vi "Dimmer BaseStation.vi"() -> ()   [LabVIEW 2014, in "ESP8266 WiFi Wrapper.lvlib"]
uses:
  ESP8266 WiFi Wrapper.lvlib
  <vilib>/Aledyne-TSXperts/Arduino Compatible Compiler for LabVIEW/Arduino Compatible Compiler for LabVIEW.lvlib
panel:
  in  "DNS address":u8[](array[numeric])=[1, 2, 3, 4]
  in  "IP address":u8[](array[numeric])=[192, 168, 0, 42]
  in  "Gateway":u8[](array[numeric])=[192, 168, 0, 1]
  in  "Subnet mask":u8[](array[numeric])=[255, 255, 255, 0]
  in  "Password":string="12345678"
  in  "SSID":string="ESP8266 Wifi Example"
  in  "Listen Port":u8=80
  in  "error in (no error)":errorcluster
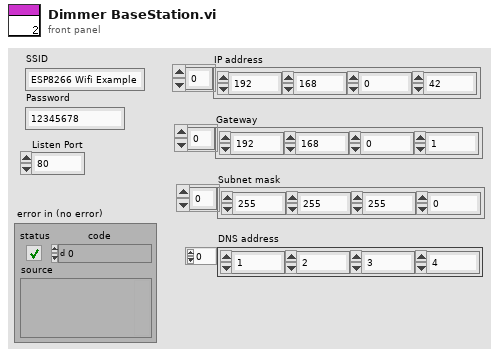
[diagram p1: front panel]
types:
  T1 = enum16{"WIFI_OFF", "WIFI_STA", "WIFI_AP", "WIFI_AP_STA"}
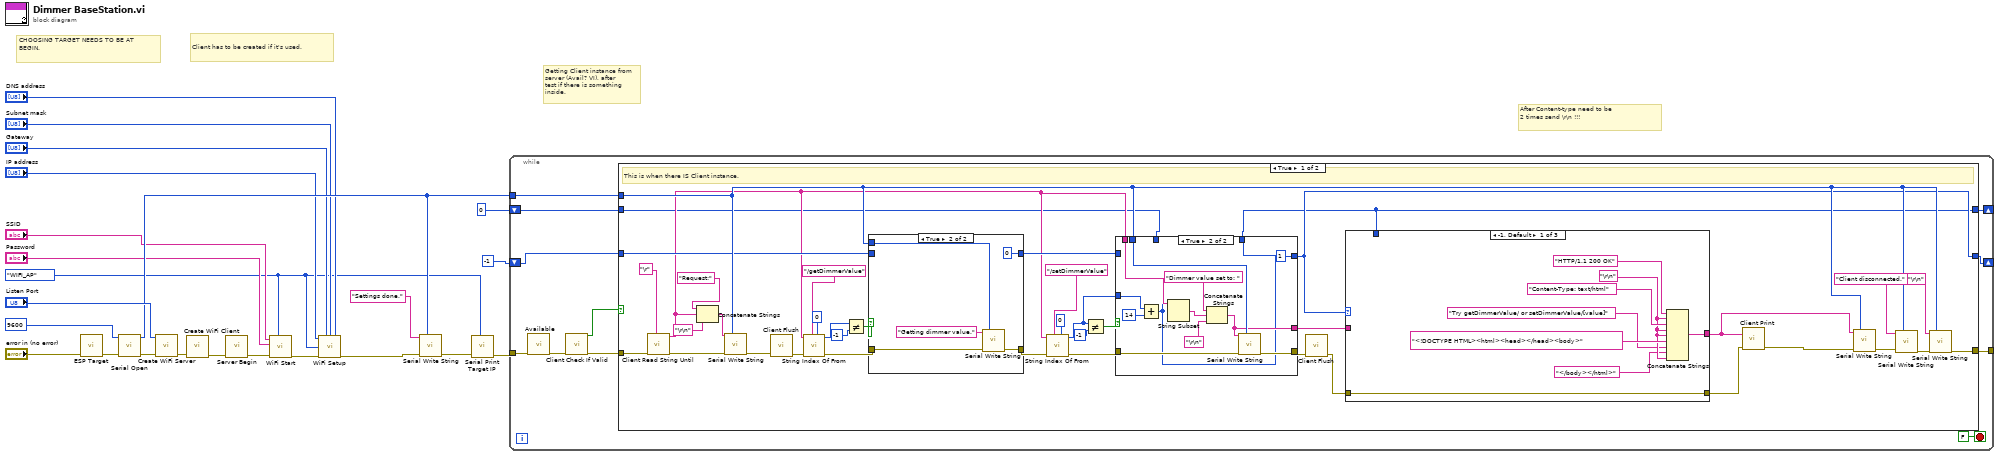
[diagram p0: block diagram]
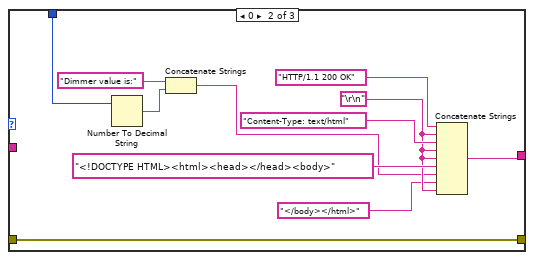
[diagram p2: hidden frame]
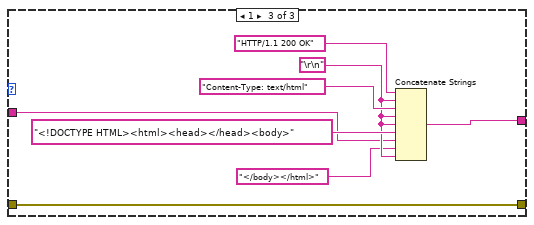
[diagram p3: hidden frame]
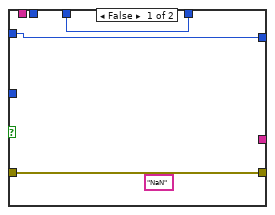
[diagram p4: hidden frame]
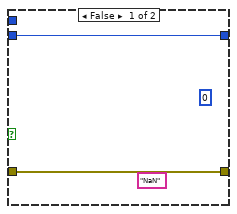
[diagram p5: hidden frame]
diagram:
  w3 = T1."WIFI_AP" ("WiFi Server Mode")
  # "After Content-type need to be\n2 times send \\r\\n !!!"
  # "Getting Client instance from\nserver (Avail? VI), after\ntest if there is something\ninside."
  # "CHOOSING TARGET NEEDS TO BE AT BEGIN."
  # "Client has to be created if it's used."
  n1 = call "ESP Target.vi"("Error In"="error in (no error)") -> ("Error Out"=w19:errorcluster)  [unwired: 10 in]
  n2 = call <vilib>:"Serial Open.vi"("Speed"=u32 9600, "error in (no error)"=w19) -> ("Instance"=w17:u8, "error out"=w22:errorcluster)  [unwired: 12 in]
  n3 = call "Create WiFi Server.vi"("Error In"=w22, "Listen Port"="Listen Port") -> ("Error Out"=w20:errorcluster)  [unwired: 9 in]
  n4 = call "Create WiFi Client.vi"("Error In"=w20) -> ("Error Out"=w13:errorcluster)  [unwired: 10 in]
  n5 = call "Server Begin.vi"("Error In"=w13) -> ("Error Out"=w15:errorcluster)  [unwired: 10 in]
  n6 = call "WiFi Start.vi"("WiFi Mode"=w3, "Error In"=w15, "Password"="Password", "SSID"="SSID") -> ("Error Out"=w14:errorcluster)  [unwired: 7 in]
  n7 = call "WiFi Setup.vi"("IP address"="IP address", "Gateway address"="Gateway", "Subnet mask"="Subnet mask", "DNS address"="DNS address", "WiFi Mode"=w3, "Error In"=w14) -> ("Error Out"=w12:errorcluster)  [unwired: 9 in]
  n8 = call <vilib>:"Serial Write String.vi"("String"="Settings done.", "Instance"=w17, "error in (no error)"=w12) -> ("error out"=w5:errorcluster)  [unwired: 12 in]
  n9 = call "Serial Print Target IP.vi"("WiFi Mode"=w3, "Error In"=w5) -> ("Error Out"=w4:errorcluster)  [unwired: 9 in]
  n10 = while {
    tunnel: [w32] -> _
    tunnel: w17 -> [w31]
    tunnel: w4 -> [w28]
    shift-right: [w27] -> _
    shift-left: i8 -1 ("Start from") -> [w26]
    shift-right: [w25] -> _
    shift-left: u8 0 ("Start from") -> [w24]
    stop <- FALSE stop-if-true
    n11 = call "Available.vi"("Error In"=w28) -> ("Error Out"=w29:errorcluster)  [unwired: 10 in]
    n12 = call "Client Check If Valid.vi"("Error In"=w29) -> ("Error Out"=w30:errorcluster, "Is Null?"=w33:bool)  [unwired: 9 in]
    n13 = case shown="True" w33 {
      tunnel: w30 -> [w73 w125]
      tunnel: [w61 w125] -> w32
      tunnel: w31 -> [w47 _]
      tunnel: w26 -> [w44 w124]
      tunnel: [w39 w124] -> w27
      tunnel: w24 -> [w37 w123]
      tunnel: [w36 w123] -> w25
      frame True {
        # "This is when there IS Client instance."
        n14 = call "Client Read String Until.vi"("Terminator char"="\r" ("Carriage Return Constant"), "Error In"=w73) -> ("Error Out"=w66:errorcluster, "Read String"=w42:string)  [unwired: 8 in]
        n15 = Concatenate Strings("Request:" ("string"), w42, "\r\n" ("End of Line Constant")) -> (w60:string)
        n16 = call <vilib>:"Serial Write String.vi"("String"=w60, "Instance"=w47, "error in (no error)"=w66) -> ("error out"=w65:errorcluster)  [unwired: 12 in]
        n17 = call "Client Flush.vi"("Error In"=w65) -> ("Error Out"=w53:errorcluster)  [unwired: 10 in]
        n18 = call "String Index Of From.vi"("Start from"=u8 0, "Find string"="/getDimmerValue" ("IndexOf String"), "Error In"=w53, "Input String"=w42) -> ("Error Out"=w52:errorcluster, "index"=w35:i8)  [unwired: 6 in]
        n19 = Not Equal?(x=w35, y=i8 -1) -> (x != y?=w71:bool)
        n20 = case shown="True" w71 {
          tunnel: [w117 w122] -> w50
          tunnel: w52 -> [w117 w121]
          tunnel: w47 -> [_ w120]
          tunnel: w44 -> [w116 _]
          tunnel: [w116 i8 0 ("Start from")] -> w43
          frame False {
            (unwired) "NaN"
            (unwired) i8 0 ("index")
          }
          frame True {
            n21 = call <vilib>:"Serial Write String.vi"("String"="Getting dimmer value.", "Instance"=w120, "error in (no error)"=w121) -> ("error out"=w122:errorcluster)  [unwired: 12 in]
          }
        }
        n22 = call "String Index Of From.vi"("Start from"=u8 0, "Find string"="/setDimmerValue" ("IndexOf String"), "Error In"=w50, "Input String"=w42) -> ("Error Out"=w49:errorcluster, "index"=w46:i8)  [unwired: 6 in]
        n23 = Not Equal?(x=w46, y=i8 -1) -> (x != y?=w68:bool)
        n24 = case shown="True" w68 {
          tunnel: [w103 w115] -> w67
          tunnel: w49 -> [w103 w113]
          tunnel: w47 -> [_ w114]
          tunnel: w46 -> [_ w110]
          tunnel: [w102 i8 1 ("Start from")] -> w39
          tunnel: w43 -> [w102 _]
          tunnel: w42 -> [_ w111]
          tunnel: [_ w105] -> w38
          tunnel: w37 -> [w101 _]
          tunnel: [w101 w104] -> w36
          frame False {
            (unwired) "NaN"
          }
          frame True {
            n25 = Add(x=w110, y=i8 14) -> (x+y=w104:i8)
            n26 = String Subset(string=w111, offset (0)=w104) -> (substring=w108:string)  [unwired: 1 in]
            n27 = Concatenate Strings("Dimmer value set to: " ("IndexOf String"), w108, "\r\n" ("End of Line Constant")) -> (w105:string)
            n28 = call <vilib>:"Serial Write String.vi"("String"=w105, "Instance"=w114, "error in (no error)"=w113) -> ("error out"=w115:errorcluster)  [unwired: 12 in]
          }
        }
        n29 = call "Client Flush.vi"("Error In"=w67) -> ("Error Out"=w41:errorcluster)  [unwired: 10 in]
        n30 = case shown="-1, Default" w39 {
          tunnel: [w75 w87 w100] -> w56
          tunnel: w41 -> [w81 w86 w96]
          tunnel: [w81 w86 w96] -> w40
          tunnel: w38 -> [_ _ w93]
          tunnel: w36 -> [_ w85 _]
          frame -1, Default {
            w77 = "\r\n" ("End of Line Constant")
            n31 = Concatenate Strings("HTTP/1.1 200 OK", w77, "Content-Type: text/html", w77, w77, "<!DOCTYPE HTML><html><head></head><body>", "Try getDimmerValue/ or setDimmerValue/[value]" ("string"), "</body></html>" ("string"), w77) -> (w75:string)
          }
          frame 0 {
            w89 = "\r\n" ("End of Line Constant")
            n32 = Number To Decimal String(number=w85) -> (decimal integer string=w84:string)  [unwired: 1 in]
            n33 = Concatenate Strings("Dimmer value is:" ("string"), w84) -> (w82:string)
            n34 = Concatenate Strings("HTTP/1.1 200 OK", w89, "Content-Type: text/html", w89, w89, "<!DOCTYPE HTML><html><head></head><body>", w82, "</body></html>" ("string"), w89) -> (w87:string)
          }
          frame 1 {
            w95 = "\r\n" ("End of Line Constant")
            n35 = Concatenate Strings("HTTP/1.1 200 OK", w95, "Content-Type: text/html", w95, w95, "<!DOCTYPE HTML><html><head></head><body>", w93, "</body></html>" ("string"), w95) -> (w100:string)
          }
        }
        n36 = call "Client Print.vi"("Error In"=w40, "Input String"=w56) -> ("Error Out"=w55:errorcluster)  [unwired: 9 in]
        n37 = call <vilib>:"Serial Write String.vi"("String"=w56, "Instance"=w47, "error in (no error)"=w55) -> ("error out"=w57:errorcluster)  [unwired: 12 in]
        n38 = call <vilib>:"Serial Write String.vi"("String"="Client disconnected.", "Instance"=w47, "error in (no error)"=w57) -> ("error out"=w64:errorcluster)  [unwired: 12 in]
        n39 = call <vilib>:"Serial Write String.vi"("String"="\r\n" ("End of Line Constant"), "Instance"=w47, "error in (no error)"=w64) -> ("error out"=w61:errorcluster)  [unwired: 12 in]
      }
      frame False {
        # "No Client instance, do nothing."
      }
    }
  }
